vi "set Volume Index And Time.vi"(8 "error in (no error)":errorcluster, 9 "pVolumeTimeInSeconds":dbl, 10 "pVolumeIndex":i32, 11 "pSinkId":i32) -> (0 "error out":errorcluster, 3 "function return":i32)   [LabVIEW 2012, in "clearvolume.lvlib"]
doc: "__declspec(dllexport) long __cdecl setVolumeIndexAndTime( long pSinkId,\n long pVolumeIndex,\n double pVolumeTimeInSeconds);"
uses:
  clearvolume.lvlib
  clearvolume.dll
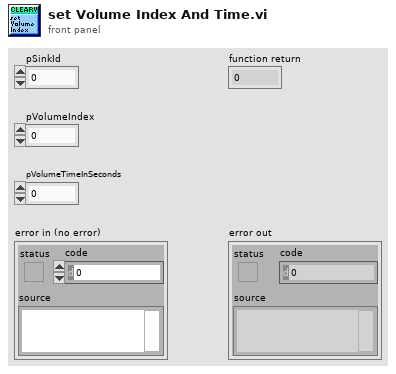
[diagram p1: front panel]
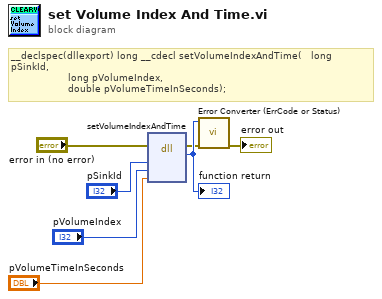
[diagram p0: block diagram]
diagram:
  # "__declspec(dllexport) long __cdecl setVolumeIndexAndTime( \t\tlong pSinkId,\n\t\t\t\t\t\t\t\t\t\t\t\t\t\t\t\t\t\t\tlong pVolumeIndex,\n\t\t\t\t\t\t\t\t\t\t\t\t\t\t\t\t\t\t\tdouble pVolumeTimeInSeconds);"
  n1 = dll-call lib="C:/Users/myerslab/workspace/Libraries/CV/clearvolume/src/labview/clearvolume/clearvolume.*" fn="setVolumeIndexAndTime"(error in="error in (no error)", "pSinkId"="pSinkId", "pVolumeIndex"="pVolumeIndex", "pVolumeTimeInSeconds"="pVolumeTimeInSeconds") -> (error out=w2:errorcluster, w7:i32)  [unwired: 5 in, 1 out]
  "function return" <- w7
  n2 = call "Error Converter (ErrCode or Status).vi"("error in (no error)"=w2, "error code"=w7) -> ("error out"=→"error out":errorcluster)  [unwired: 9 in]
